vi "True Symbol Image Constant.vi"() -> (1 "True Symbol Image Contant":T1={"image type"=0, "image depth"=24, "image"=[142, 143, 143, 142, 143, 143, 142, 143, 143, 142, 143, 143, 142, 143, 143, 142, 143, 143, 142, 143, 143, 142, 143, 143, 142, 143, 143, 142, 143, 143, 142, 143, 143, 142, 143, 143, 142, 143, 143, 142, 143, 143, 244, 244, 244, 244, 244, 244, 244, 244, 244, 244, 244, 244, 244, 244, 244, 244, 244, 244, 244, 244, 244, 244, 244, 244, 244, 244, 244, 244, 244, 244, 244, 244, 244, 142, 143, 143, 142, 143, 143, 244, 244, 244, 174, 179, 185, 174, 179, 185, 174, 179, 185, 174, 179, 185, 174, 179, 185, 174, 179, 185, 175, 180, 186, 180, 185, 189, 187, 190, 193, 244, 244, 244, 142, 143, 143, 142, 143, 143, 244, 244, 244, 174, 179, 185, 203, 207, 213, 203, 207, 213, 203, 207, 213, 203, 207, 213, 208, 211, 216, 213, 216, 220, 219, 221, 223, 193, 195, 197, 244, 244, 244, 142, 143, 143, 142, 143, 143, 244, 244, 244, 174, 179, 185, 203, 207, 213, 203, 207, 213, 205, 209, 214, 210, 213, 218, 216, 219, 222, 221, 223, 225, 226, 227, 228, 198, 199, 200, 244, 244, 244, 142, 143, 143, 142, 143, 143, 244, 244, 244, 174, 179, 185, 205, 209, 215, 208, 212, 217, 212, 215, 219, 219, 221, 223, 225, 226, 227, 229, 230, 230, 232, 232, 232, 204, 205, 205, 244, 244, 244, 142, 143, 143, 142, 143, 143, 244, 244, 244, 178, 183, 188, 213, 216, 220, 218, 220, 223, 224, 225, 227, 232, 232, 232, 236, 236, 236, 237, 237, 237, 237, 237, 237, 212, 213, 214, 244, 244, 244, 142, 143, 143, 142, 143, 143, 244, 244, 244, 184, 187, 191, 221, 223, 225, 228, 229, 229, 234, 234, 234, 239, 239, 239, 242, 242, 242, 242, 242, 242, 242, 242, 242, 220, 221, 222, 244, 244, 244, 142, 143, 143, 142, 143, 143, 244, 244, 244, 188, 191, 194, 227, 228, 229, 233, 233, 233, 237, 237, 237, 242, 242, 242, 244, 244, 244, 245, 245, 245, 244, 244, 244, 225, 226, 226, 244, 244, 244, 142, 143, 143, 142, 143, 143, 244, 244, 244, 194, 196, 198, 233, 233, 233, 237, 237, 237, 240, 240, 240, 244, 244, 244, 246, 246, 246, 246, 246, 246, 246, 246, 246, 230, 230, 230, 244, 244, 244, 142, 143, 143, 142, 143, 143, 244, 244, 244, 202, 203, 204, 212, 212, 213, 219, 219, 220, 224, 225, 225, 230, 231, 231, 234, 235, 235, 235, 236, 236, 235, 235, 236, 233, 233, 234, 244, 244, 244, 142, 143, 143, 142, 143, 143, 244, 244, 244, 244, 244, 244, 244, 244, 244, 244, 244, 244, 244, 244, 244, 244, 244, 244, 244, 244, 244, 244, 244, 244, 244, 244, 244, 244, 244, 244, 244, 244, 244, 142, 143, 143, 142, 143, 143, 142, 143, 143, 142, 143, 143, 142, 143, 143, 142, 143, 143, 142, 143, 143, 142, 143, 143, 142, 143, 143, 142, 143, 143, 142, 143, 143, 142, 143, 143, 142, 143, 143, 142, 143, 143], "mask"=[], "colors"=[], "Rectangle"={"left"=0, "top"=0, "right"=13, "bottom"=13}})   [LabVIEW 2015, in "MulticolumnListboxSelection.lvclass"]
doc: "<b> </b> <b> </b>\n©2016 Q Software Innovations, LLC (QSI)\nwritten by Quentin Alldredge\nproduced in LabVIEW 2015\n\nsupport@qsoftwareinnovations.com\nwww.qsoftwareinnovations.com\n\nAll rights reserved.\n\nRedistribution and use in source and binary forms, with or without modification, are permitted provided that the following conditions are met:\n\n * Redistributions of source code must retain the above copyright notice, this list of conditions and the following disclaimer.\n * Redistributions in binary form must reproduce the above copyright notice, this list of conditions and the following disclaimer in the documentation and/or other materials provided with the distribution.\n * Neither the name of Q Software Innovations, LLC. nor the names of its contributors may be used to endorse or promote products derived from this software without specific prior written permission.\n\nTHIS SOFTWARE IS PROVIDED BY THE COPYRIGHT HOLDERS AND CONTRIBUTORS \"AS IS\" AND ANY EXPRESS OR IMPLIED WARRANTIES, INCLUDING, BUT NOT LIMITED TO, THE IMPLIED WARRANTIES OF MERCHANTABILITY AND FITNESS FOR A PARTICULAR PURPOSE ARE DISCLAIMED. IN NO EVENT SHALL THE COPYRIGHT OWNER OR CONTRIBUTORS BE LIABLE FOR ANY DIRECT, INDIRECT, INCIDENTAL, SPECIAL, EXEMPLARY, OR CONSEQUENTIAL DAMAGES (INCLUDING, BUT NOT LIMITED TO, PROCUREMENT OF SUBSTITUTE GOODS OR SERVICES; LOSS OF USE, DATA, OR PROFITS; OR BUSINESS INTERRUPTION) HOWEVER CAUSED AND ON ANY THEORY OF LIABILITY, WHETHER IN CONTRACT, STRICT LIABILITY, OR TORT (INCLUDING NEGLIGENCE OR OTHERWISE) ARISING IN ANY WAY OUT OF THE USE OF THIS SOFTWARE, EVEN IF ADVISED OF THE POSSIBILITY OF SUCH DAMAGE."
uses:
  MulticolumnListboxSelection.lvclass
  <vilib>/picture/picture.llb/imagedata.ctl
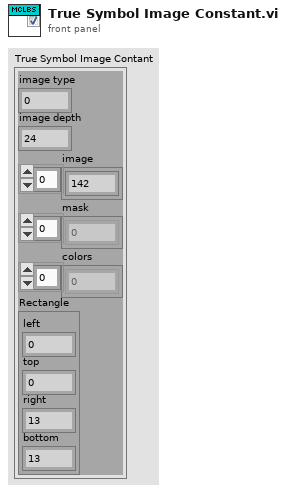
[diagram p1: front panel]
types:
  T1 = typedef "imagedata.ctl" = cluster{"image type":i32, "image depth":i32, "image":u8[], "mask":u8[], "colors":u32[], "Rectangle":cluster{"left":i16, "top":i16, "right":i16, "bottom":i16}}
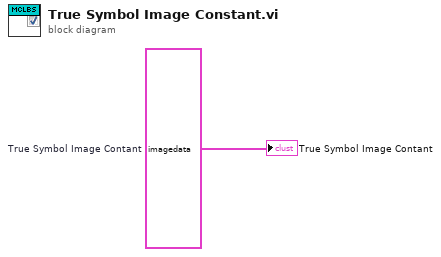
[diagram p0: block diagram]
diagram:
  w1 = T1 {"image type"=0, "image depth"=24, "image"=[142, 143, 143, 142, 143, 143, 142, 143, 143, 142, 143, 143, 142, 143, 143, 142, 143, 143, 142, 143, 143, 142, 143, 143, 142, 143, 143, 142, 143, 143, 142, 143, 143, 142, 143, 143, 142, 143, 143, 142, 143, 143, 244, 244, 244, 244, 244, 244, 244, 244, 244, 244, 244, 244, 244, 244, 244, 244, 244, 244, 244, 244, 244, 248, 248, 248, 249, 249, 249, 246, 246, 246, 244, 244, 244, 142, 143, 143, 142, 143, 143, 244, 244, 244, 174, 179, 185, 174, 179, 185, 174, 179, 185, 174, 179, 185, 174, 179, 185, 201, 204, 208, 157, 167, 192, 119, 134, 171, 220, 223, 228, 245, 245, 245, 142, 143, 143, 142, 143, 143, 244, 244, 244, 174, 179, 185, 203, 207, 213, 203, 207, 213, 203, 207, 213, 204, 208, 214, 237, 238, 241, 87, 106, 157, 68, 90, 146, 185, 191, 208, 246, 246, 246, 142, 143, 143, 142, 143, 143, 244, 244, 244, 174, 179, 185, 203, 207, 213, 203, 207, 213, 205, 209, 214, 224, 226, 230, 175, 184, 207, 69, 90, 146, 101, 119, 165, 231, 231, 232, 244, 244, 244, 142, 143, 143, 142, 143, 143, 244, 244, 244, 174, 179, 185, 213, 217, 221, 223, 226, 229, 213, 216, 220, 242, 243, 244, 94, 113, 161, 71, 92, 148, 188, 195, 214, 219, 220, 220, 244, 244, 244, 142, 143, 143, 142, 143, 143, 244, 244, 244, 197, 201, 205, 201, 207, 221, 163, 174, 200, 237, 238, 238, 186, 193, 213, 73, 94, 150, 100, 118, 165, 248, 248, 248, 213, 213, 214, 244, 244, 244, 142, 143, 143, 142, 143, 143, 244, 244, 244, 222, 224, 225, 110, 127, 170, 71, 92, 148, 207, 212, 226, 103, 120, 167, 75, 96, 151, 183, 191, 213, 246, 246, 246, 220, 221, 222, 244, 244, 244, 142, 143, 143, 142, 143, 143, 244, 244, 244, 205, 207, 209, 222, 225, 233, 72, 93, 149, 73, 95, 150, 75, 96, 151, 97, 115, 164, 248, 249, 250, 244, 244, 244, 225, 226, 226, 244, 244, 244, 142, 143, 143, 142, 143, 143, 244, 244, 244, 198, 200, 202, 234, 236, 240, 139, 153, 187, 74, 95, 151, 76, 97, 152, 176, 185, 209, 249, 249, 249, 246, 246, 246, 230, 230, 230, 244, 244, 244, 142, 143, 143, 142, 143, 143, 244, 244, 244, 202, 203, 204, 218, 218, 219, 223, 226, 233, 140, 153, 186, 144, 157, 189, 242, 243, 246, 236, 237, 237, 235, 235, 236, 233, 233, 234, 244, 244, 244, 142, 143, 143, 142, 143, 143, 244, 244, 244, 244, 244, 244, 244, 244, 244, 245, 245, 245, 249, 249, 249, 248, 248, 248, 245, 245, 245, 244, 244, 244, 244, 244, 244, 244, 244, 244, 244, 244, 244, 142, 143, 143, 142, 143, 143, 142, 143, 143, 142, 143, 143, 142, 143, 143, 142, 143, 143, 142, 143, 143, 142, 143, 143, 142, 143, 143, 142, 143, 143, 142, 143, 143, 142, 143, 143, 142, 143, 143, 142, 143, 143], "mask"=[], "colors"=[], "Rectangle"={"left"=0, "top"=0, "right"=13, "bottom"=13}}  # True Symbol Image Contant
  "True Symbol Image Contant" <- w1
